vi "Pose.vi"() -> ()   [LabVIEW 2016]
panel:
  out "Lidar Directions":dbl[](array[numeric])
  out "Lidar Magnitudes":dbl[](array[numeric])
  in  "Bot Angle":dbl
  in  "Wall Angle":dbl
  in  "Wall Distance":dbl
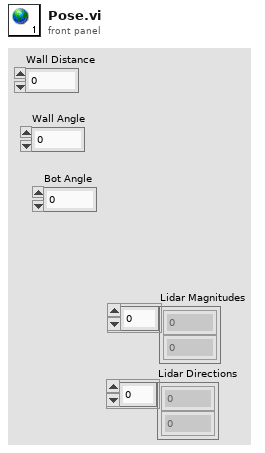
[diagram p1: front panel]
diagram:
